vi "Modbus_facory.vi"() -> ()   [LabVIEW 2020]
uses:
  <vilib>/NI/Modbus Library/API/Wrapper/Create TCP Master.vi
  <vilib>/ErrorRing/Error Ring.xnode
  <vilib>/NI/Modbus Library/API/Master/Modbus Master.lvclass
  <vilib>/NI/Modbus Library/API/Wrapper/API Main.lvlib
panel:
  in  "Stop2":bool
  in  "Faja4":bool
  in  "Faja 2":bool
  in  "Stop1":bool
  in  "Faja3":bool
  in  "Faja 1":bool
  in  "valvula de descarga":u16(slide) scale=0.0..10.0
  in  "Valvula de carga":u16(slide) scale=0.0..10.0
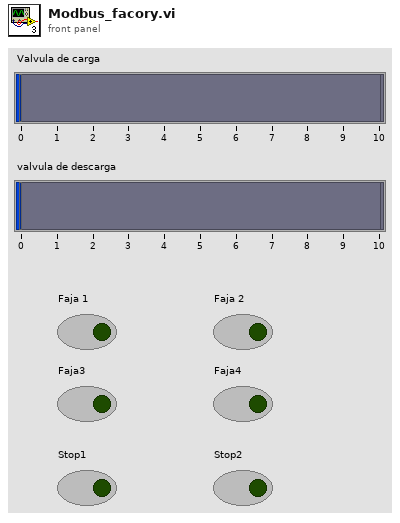
[diagram p1: front panel]
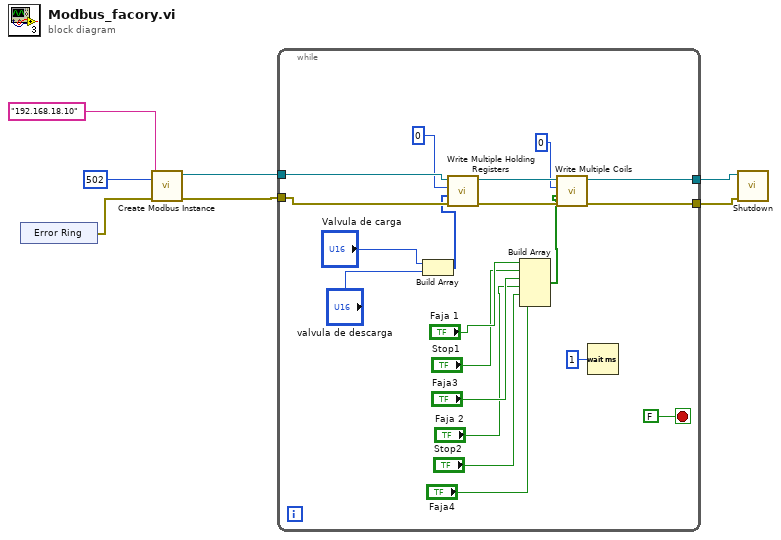
[diagram p0: block diagram]
diagram:
  n1 = xnode "Error Ring"() -> ("error out"=w5:errorcluster)
  n2 = call-poly <vilib>:"Create Modbus Instance.vi"("error in"=w5, "port (502)"=u16 502, "address"="192.168.18.10") -> ("error out"=w3:errorcluster, "TCP master instance"=w4:refnum<class "Modbus Master.lvclass">)  [unwired: 7 in]
  n3 = while {
    tunnel: w4 -> [w26]
    tunnel: w3 -> [w25]
    tunnel: [w18] -> w2
    tunnel: [w17] -> w1
    stop <- FALSE stop-if-true
    n4 = Build Array("Valvula de carga", "valvula de descarga") -> (w20:u16[])
    n5 = call-dynamic "Write Multiple Holding Registers.vi"("error in"=w25, "registers to write"=w20, "starting address"=u16 0, "Modbus master in"=w26) -> ("error out"=w16:errorcluster, "Modbus master out"=w19:refnum<class "Modbus Master.lvclass">)  [unwired: 6 in]
    n6 = Build Array("Faja 1", "Stop1", "Faja3", "Faja 2", "Stop2", "Faja4") -> (w15:bool[])
    n7 = call-dynamic "Write Multiple Coils.vi"("error in"=w16, "coils to write"=w15, "starting address"=u16 0, "Modbus master in"=w19) -> ("error out"=w17:errorcluster, "Modbus master out"=w18:refnum<class "Modbus Master.lvclass">)  [unwired: 6 in]
    n8 = Wait (ms)(milliseconds to wait=u32 1) -> ()  [unwired: 1 out]
  }
  n9 = call-dynamic "Shutdown.vi"("error in"=w1, "Modbus master in"=w2) -> ()  [unwired: 9 in, 1 out]
